vi "Test WMI Battery Status.vi"() -> ()   [LabVIEW 2012]
panel:
  out "Numeric":i32
  out "estRT":i32
  out "Status":string
  in  "Boolean":bool
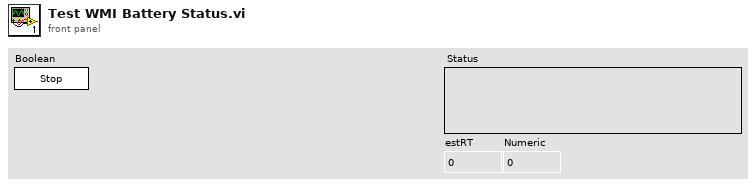
[diagram p1: front panel]
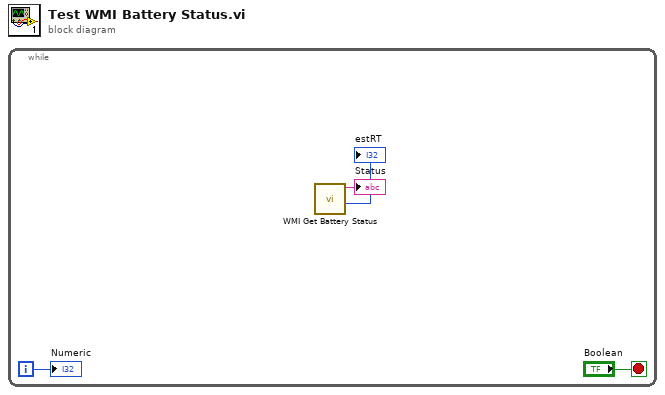
[diagram p0: block diagram]
diagram:
  n1 = while {
    i -> [w1]
    stop <- "Boolean" stop-if-true
    n2 = call "WMI Get Battery Status.vi"() -> ("estRT"=→"estRT":i32, "Status"=→"Status":string)  [unwired: 8 in, 2 out]
    "Numeric" <- w1
  }
